vi "Compute Optimal Transition Time.vi"(8 "error in (no error)":errorcluster, 10 "optimum":T1, 11 "SV Continuous Sweep in":refnum<class "SV Continuous Sweep.lvclass">) -> (0 "error out":errorcluster, 2 "optimal transition time":dbl, 3 "SV Continuous Sweep out":refnum<class "SV Continuous Sweep.lvclass">)   [LabVIEW 2017, in "SV Continuous Sweep.lvclass"]
uses:
  <vilib>/addons/_NISVFA/_Generation/Signal Generation/SV Continuous Sweep/SV Continuous Sweep.lvclass
  C:/Program Files (x86)/National Instruments/LabVIEW 2017/vi.lib/addons/_NISVFA/_Generation/Signal Generation/SV Signal/SV Signal.lvclass
  <vilib>/addons/_NISVFA/_Generation/subVIs/sv_Optimum Location.ctl
  <vilib>/addons/_NISVFA/_Generation/Signal Generation/SV Signal/sv_Signal State Attribute.ctl
  <vilib>/addons/_NISVFA/_Generation/Signal Generation/SV Continuous Sweep/SV Continuous Sweep.lvclass/SV Continuous Sweep.ctl
  <vilib>/addons/_NISVFA/_Generation/Signal Generation/SV Signal/Read Sample Rate.vi
  <vilib>/addons/_NISVFA/_Generation/Signal Generation/SV Signal/SV Signal.lvclass
  <vilib>/addons/_NISVFA/_Generation/SoundVib_Generation.lvlib
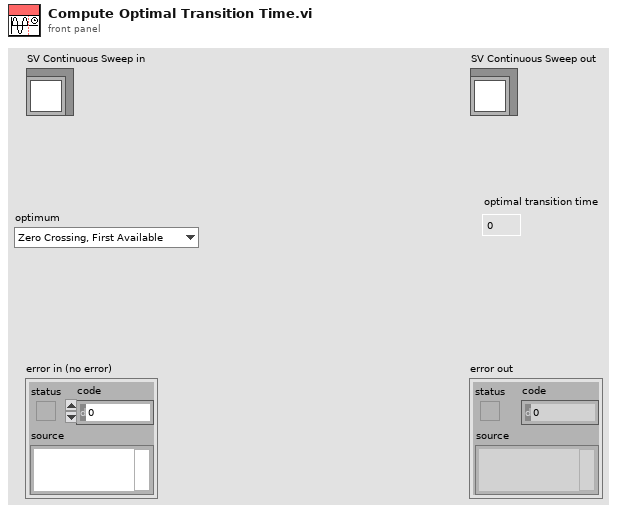
[diagram p1: front panel]
types:
  T1 = typedef "SoundVib_Generation.lvlib/sv_Optimum Location.ctl" = enum16{"Zero Crossing, First Available", "Zero Crossing, Positive Slope", "Zero Crossing, Negative Slope", "Peak or Valley", "Peak", "Valley"}
  T2 = typedef "SV Signal.lvclass/sv_Signal State Attribute.ctl" = string
  T3 = typedef "SV Signal.lvclass/sv_System Timing Model.ctl" = i64
  T4 = typedef "SV Signal.lvclass/sv_Generation State.ctl" = enum16{"Idle", "Ramp Up", "Pre-Measurement Settling", "Measurement", "Post-Measurement Settling", "Discrete Sweep Transition", "Ramp Down", "Update"}
  T5 = cluster{"system timing model":T3, "state":cluster{"RESET":bool, "generator timestamp":timestamp, "elapsed seconds":dbl, "elapsed samples":u64, "generation state":T4, "time offset at state":dbl, "samples generated at state":u64, "signal state":variant}, "duration of state":dbl, "samples remaining at state":i32}
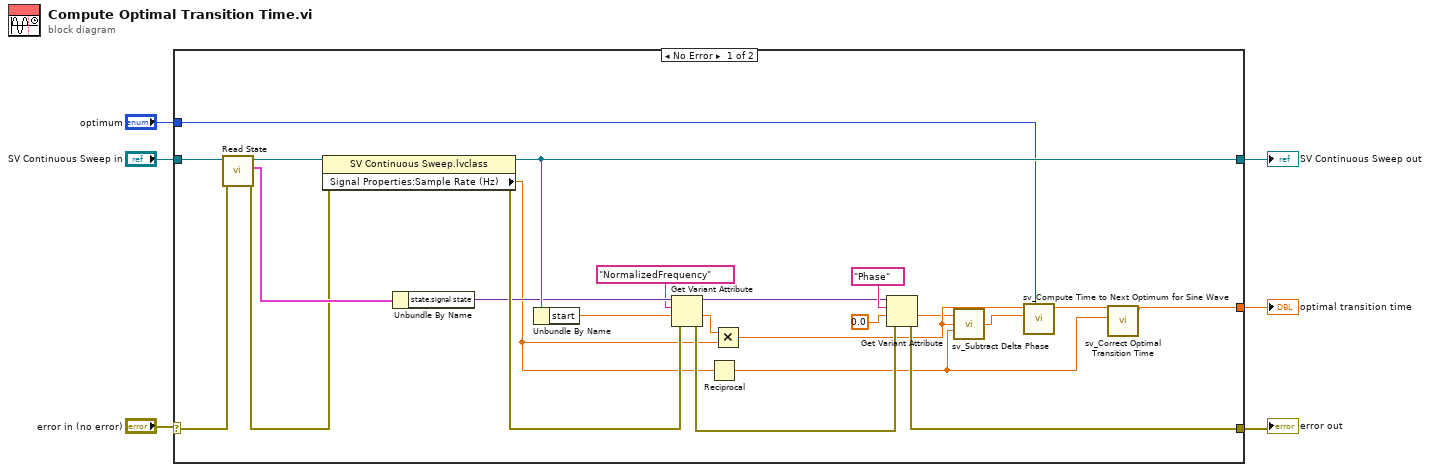
[diagram p0: block diagram]
diagram:
  n1 = case shown="No Error" "error in (no error)" {
    selector: "error in (no error)" -> [w24 w32]
    tunnel: [w29 w32] -> w5
    tunnel: [w30 w31] -> w4
    tunnel: "SV Continuous Sweep in" -> [w27 w31]
    tunnel: [w8 _] -> w2
    tunnel: "optimum" -> [w21 _]
    frame No Error {
      n2 = call <vilib>:"Read State.vi"("error in (no error)"=w24, "signal configuration"=w27) -> ("error out"=w23:errorcluster, "generator state"=w25:T5, "signal configuration"=w26:refnum<class "SV Continuous Sweep.lvclass">)  [unwired: 7 in]
      n3 = property class="SV Continuous Sweep.lvclass"(reference=w26, error in=w23) -> (reference out=w30:refnum<class "SV Continuous Sweep.lvclass">, error out=w28:errorcluster, "Signal Properties:Sample Rate (Hz)"=w13:dbl)
      n4 = Unbundle By Name(w25) -> ("state.signal state"=w22:variant)
      n5 = Unbundle By Name(w30) -> ("start"=w17:dbl)
      n6 = Get Variant Attribute(Variant=w22, name=T2 "NormalizedFrequency", default value (empty Variant)=w17, error in=w28) -> (duplicate Variant=w15:variant, value=w16:dbl, error out=w14:errorcluster)  [unwired: 1 out]
      n7 = Reciprocal(x=w13) -> (1/x=w7:dbl)
      n8 = Multiply(x=w16, y=w13) -> (x*y=w12:dbl)
      n9 = Get Variant Attribute(Variant=w15, name=T2 "Phase", default value (empty Variant)=0.0 ("f"), error in=w14) -> (value=w11:dbl, error out=w29:errorcluster)  [unwired: 2 out]
      n10 = call <vilib>:"sv_Subtract Delta Phase.vi"("phase in [deg]"=w11, "frequency [Hz]"=w12, "dt [s]"=w7) -> ("phase out [deg]"=w10:dbl)  [unwired: 12 in]
      n11 = call <vilib>:"sv_Compute Time to Next Optimum for Sine Wave.vi"("optimum"=w21, "phase (0 °)"=w10, "frequency (997 Hz)"=w12) -> ("time to optimum [s]"=w9:dbl)  [unwired: 8 in]
      n12 = call <vilib>:"sv_Correct Optimal Transition Time.vi"("dt"=w7, "time to optimum [s]"=w9) -> ("corrected time to optimum [s]"=w8:dbl)  [unwired: 9 in]
    }
    frame Error {
    }
  }
  "error out" <- w5
  "SV Continuous Sweep out" <- w4
  "optimal transition time" <- w2
